vi "HEWH Calculate Draw Stats.vi"(7 "Headers":string[](array[string])=["Voltage (Volts) - Mean", "Voltage (Volts) - Standard Deviation", "Voltage (Volts) - Variance", "Voltage (Volts) - Max", "Voltage (Volts) - Min", "Current (Amps) - Mean", "Current (Amps) - Standard Deviation", "Current (Amps) - Variance", "Current (Amps) - Max", "Current (Amps) - Min", "Power (Watts) - Mean", "Power (Watts) - Standard Deviation", "Power (Watts) - Variance", "Power (Watts) - Max", "Power (Watts) - Min", "", "", "", "WattHours - Max", "WattHours - Min", "TC Tree (AVG) - Mean", "TC Tree (AVG) - Standard Deviation", "TC Tree (AVG) - Variance", "TC Tree (AVG) - Max", "TC Tree (AVG) - Min", "Flow Rate (GPM) - Mean", "Flow Rate (GPM) - Standard Deviation", "Flow Rate (GPM) - Variance", "Flow Rate (GPM) - Max", "Flow Rate (GPM) - Min", "", "", "", "Gallons (Gal) - Max", "Gallons (Gal) - Min", "RTD Out (°F) - Mean", "RTD Out (°F) - Standard Deviation", "RTD Out (°F) - Variance", "RTD Out (°F) - Max", "RTD Out (°F) - Min", "RTD In (°F) - Mean", "RTD In (°F) - Standard Deviation", "RTD In (°F) - Variance", "RTD In (°F) - Max", "RTD In (°F) - Min", "RTD Ambinet (°F) - Mean", "RTD Ambient (°F) - Standard Deviation", "RTD Ambinent (°F) - Variance", "RTD Ambinent (°F) - Max", "RTD Ambinent (°F) - Min", "TC Down (°F) - Mean", "TC Down (°F) - Standard Deviation", "TC Down (°F) - Variance", "TC Down (°F) - Max", "TC Down (°F) - Min", "TC1 (°F) - Mean", "TC1 (°F) - Standard Deviation", "TC1 (°F) - Variance", "TC1 (°F) - Max", "TC1 (°F) - Min", "TC2 (°F) - Mean", "TC2 (°F) - Standard Deviation", "TC2 (°F) - Variance", "TC2 (°F) - Max", "TC2 (°F) - Min", "TC3 (°F) - Mean", "TC3 (°F) - Standard Deviation", "TC3 (°F) - Variance", "TC3 (°F) - Max", "TC3 (°F) - Min", "TC4 (°F) - Mean", "TC4 (°F) - Standard Deviation", "TC4 (°F) - Variance", "TC4 (°F) - Max", "TC4 (°F) - Min", "TC5 (°F) - Mean", "TC5 (°F) - Standard Deviation", "TC5 (°F) - Variance", "TC5 (°F) - Max", "TC5 (°F) - Min", "TC6 (°F) - Mean", "TC6 (°F) - Standard Deviation", "TC6 (°F) - Variance", "TC6 (°F) - Max", "TC6 (°F) - Min", "", "", "", "Total Harmonic Distortion (%V) - Max", "Total Harmonic Distortion (%V) - Min", "Frequency (Hz) - Mean ", "Frequency (Hz) - Standard Deviation", "Frequency (Hz) - Variance", "Frequency (Hz) - Max", "Frequency (Hz) - Min", "Apparent Power (VA) - Mean", "Apparent Power (VA) - Standard Deviation", "Apparent Power (VA) - Variance", "Apparent Power (VA) - Max", "Apparent Power (VA) - Min", "", "", "", "Power Factor - Max", "Power Factor - Min", "", "", "", "Current Crest Factor - Max", "Current Crest Factor - Min", "", "", "", "Voltage Crest Factor - Max", "Voltage Crest Factor - Min", "", "", "", "Elapsed Time (Sec) - Max", "Elapsed Time (Sec) - Min"], 8 "Error In":errorcluster, 11 "Draw Stats":dbl[][](array[numeric])) -> (0 "Error Out":errorcluster, 2 "Data With Headers":string[][](array[string]), 3 "Draw Stats Out":dbl[][](array[numeric]))   [LabVIEW 2020]
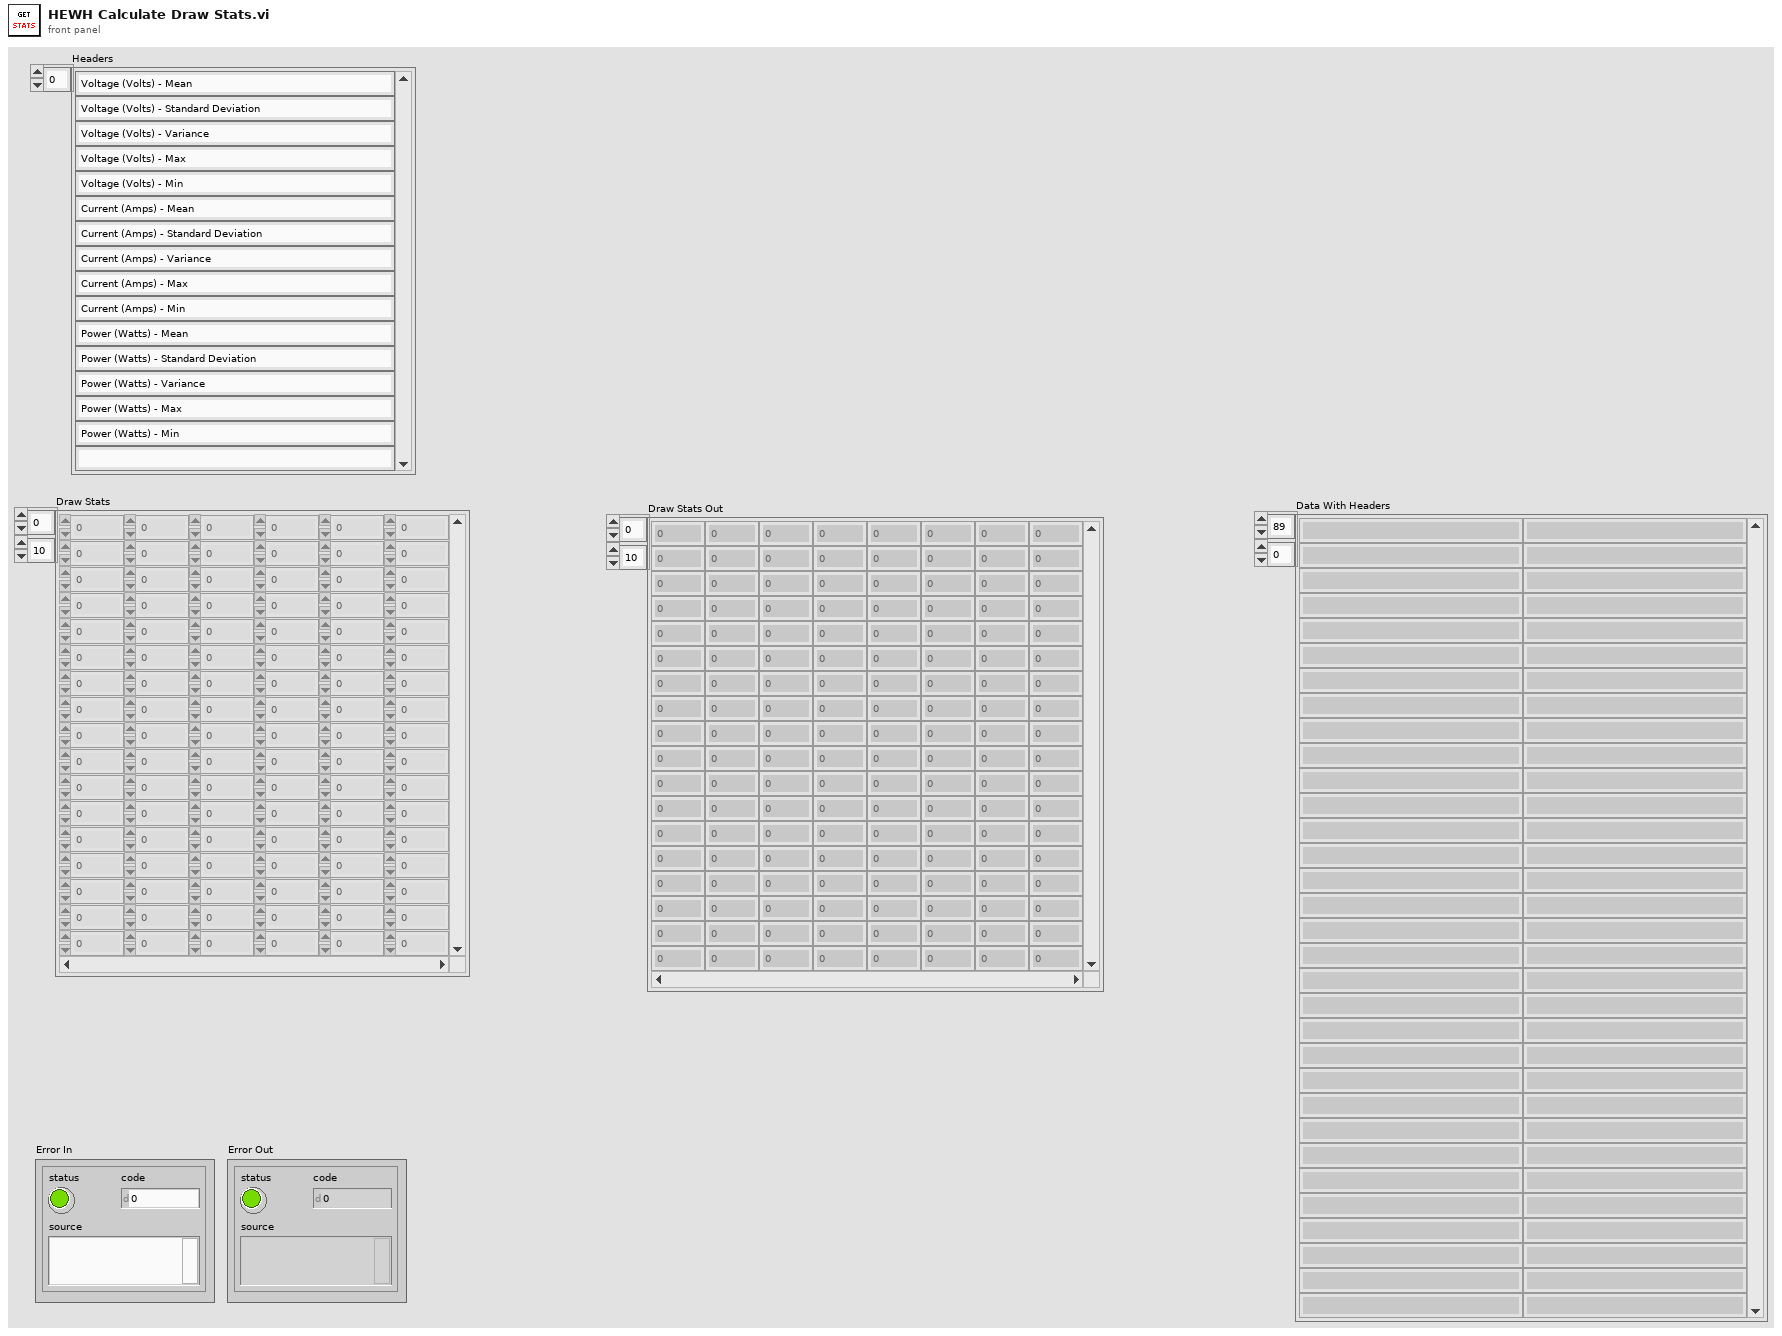
[diagram p1: front panel]
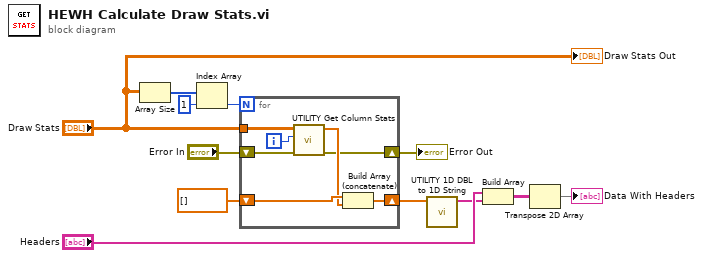
[diagram p0: block diagram]
diagram:
  n1 = Array Size(array="Draw Stats") -> (size(s)=w9:i32[])
  n2 = Index Array(array=w9, index=1) -> (element=w11:i32)
  n3 = for {
    N: w11 -> [_]
    tunnel: "Draw Stats" -> [w19]
    shift-right: [w16] -> w5
    shift-left: dbl[] [] -> [w17]
    shift-right: [w13] -> w6
    shift-left: "Error In" -> [w14]
    i -> [w18]
    n4 = call "UTILITY Get Column Stats.vi"("Error In"=w14, "Index"=w18, "Draw Stats"=w19) -> ("Error Out"=w13:errorcluster, "Column Stats"=w15:dbl[])  [unwired: 7 in]
    n5 = Build Array (concatenate)(w17, w15) -> (w16:dbl[])
  }
  "Error Out" <- w6
  n6 = call "UTILITY 1D DBL to 1D String.vi"("1D DBL"=w5) -> ("1D String"=w3:string[])  [unwired: 10 in]
  n7 = Build Array("Headers", w3) -> (w2:string[][])
  n8 = Transpose 2D Array(2D array=w2) -> (transposed array=→"Data With Headers":string[][])
  "Draw Stats Out" <- "Draw Stats"
